vi "AgNA_SetAttributeViReal64.vi"(7 "AttributeValue":dbl, 8 "error in (no error)":errorcluster {"code" format="%.0x"}, 9 "AttributeID":u32(ring)=1150004 items=["CHANNEL_CW_FREQUENCY"=1150004, "CHANNEL_IF_BANDWIDTH"=1150005, "CHANNEL_MEASUREMENT_ELECTRICAL_DELAY_DISTANCE"=1150177, "CHANNEL_MEASUREMENT_ELECTRICAL_DELAY_TIME"=1150176, "CHANNEL_MEASUREMENT_ELECTRICAL_DELAY_VELOCITY_FACTOR"=1150180, "CHANNEL_MEASUREMENT_ELECTRICAL_DELAY_WAVE_GUIDE_CUT_OFF_FREQ"=1150179, "CHANNEL_MEASUREMENT_GROUP_DELAY_FREQUENCY"=1150172, "CHANNEL_MEASUREMENT_GROUP_DELAY_PERCENT"=1150174, "CHANNEL_MEASUREMENT_GROUP_DELAY_POINTS"=1150173, "CHANNEL_MEASUREMENT_MARKER_BANDWIDTH_THRESHOLD"=1150021, "CHANNEL_MEASUREMENT_MARKER_PEAK_EXCURSION"=1150024, "CHANNEL_MEASUREMENT_MARKER_STIMULUS"=1150025, "CHANNEL_MEASUREMENT_MARKER_TARGET_VALUE"=1150026, "CHANNEL_MEASUREMENT_SMOOTHING_APERTURE"=1150016, "CHANNEL_MEASUREMENT_TIME_DOMAIN_GATING_CENTER"=1150138, "CHANNEL_MEASUREMENT_TIME_DOMAIN_GATING_SPAN"=1150141, "CHANNEL_MEASUREMENT_TIME_DOMAIN_GATING_START"=1150142, "CHANNEL_MEASUREMENT_TIME_DOMAIN_GATING_STOP"=1150143, "CHANNEL_MEASUREMENT_TIME_DOMAIN_TRANSFORM_CENTER"=1150145, "CHANNEL_MEASUREMENT_TIME_DOMAIN_TRANSFORM_SPAN"=1150148, "CHANNEL_MEASUREMENT_TIME_DOMAIN_TRANSFORM_START"=1150149, "CHANNEL_MEASUREMENT_TIME_DOMAIN_TRANSFORM_STEP_RISE_TIME"=1150150, "CHANNEL_MEASUREMENT_TIME_DOMAIN_TRANSFORM_STOP"=1150151, "CHANNEL_MEASUREMENT_TIME_DOMAIN_WINDOW_IMPULSE_WIDTH"=1150152, "CHANNEL_MEASUREMENT_TIME_DOMAIN_WINDOW_KAISER_BETA"=1150153, "CHANNEL_MEASUREMENT_TRACE_REFERENCE_POSITION"=1150027, "CHANNEL_MEASUREMENT_TRACE_REFERENCE_VALUE"=1150028, "CHANNEL_MEASUREMENT_TRACE_Y_SCALE"=1150029, "CHANNEL_STIMULUS_RANGE_CENTER"=1150032, "CHANNEL_STIMULUS_RANGE_SPAN"=1150033, "CHANNEL_STIMULUS_RANGE_START"=1150034, "CHANNEL_STIMULUS_RANGE_STOP"=1150035, "CHANNEL_SWEEP_TIME"=1150010, "GUIDED_CALIBRATION__ADVANCED_IF_BAND_WIDTH"=1150171], 10 "RepCapIdentifier":string, 11 "instrument handle":refnum<k15>) -> (0 "error out":errorcluster {"code" format="%.0x"}, 3 "instrument handle out":refnum<k15>)   [LabVIEW 2015]
uses:
  <instrlib>/Agilent NA/Agilent NA.lvlib
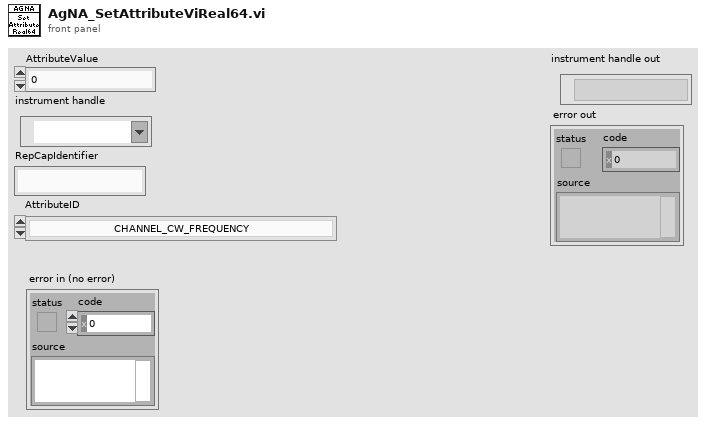
[diagram p1: front panel]
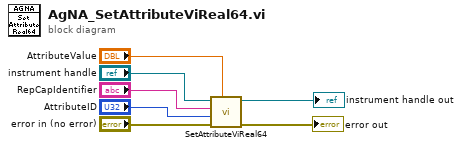
[diagram p0: block diagram]
diagram:
  n1 = call <instrlib>:"SetAttributeViReal64.vi"("AttributeValue"="AttributeValue", "error in (no error)"="error in (no error)", "AttributeID"="AttributeID", "RepCapIdentifier"="RepCapIdentifier", "instrument handle"="instrument handle") -> ("error out"=→"error out":errorcluster, "instrument handle out"=→"instrument handle out":refnum<k15>)  [unwired: 5 in]
